vi "Handle Value.vi"(8 "error in (no error)":errorcluster, 10 "Value":string, 11 "Multipart Parser in":refnum<class "Multipart Parser.lvclass">) -> (0 "error out":errorcluster, 3 "Multipart Parser out":refnum<class "Multipart Parser.lvclass">)   [LabVIEW 2020, in "HTTP Utils.lvlib" / "Multipart Parser.lvclass"]
uses:
  Multipart Parser.lvclass
  Multipart Parser.lvclass/Multipart Parser.ctl
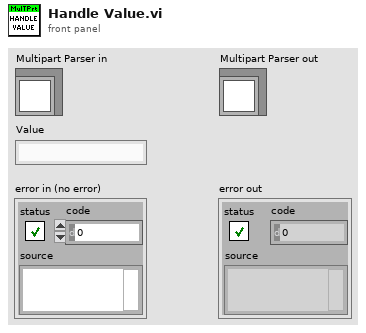
[diagram p1: front panel]
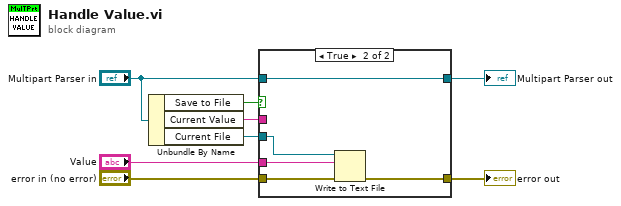
[diagram p0: block diagram]
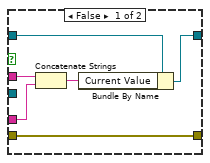
[diagram p2: hidden frame]
diagram:
  n1 = Unbundle By Name("Multipart Parser in") -> ("Save to File"=w7:bool, "Current Value"=w1:string, "Current File"=w5:refnum<file>)
  n2 = case shown="True" w7 {
    tunnel: "error in (no error)" -> [w14 w19]
    tunnel: "Value" -> [w12 w18]
    tunnel: w5 -> [_ w17]
    tunnel: [w14 w16] -> w4
    tunnel: "Multipart Parser in" -> [w11 w15]
    tunnel: [w9 w15] -> w2
    tunnel: w1 -> [w13 _]
    frame False {
      n3 = Concatenate Strings(w13, w12) -> (w10:string)
      n4 = Bundle By Name(cluster=w11, "Current Value"=w10) -> (w9:refnum<class "Multipart Parser.lvclass">)
    }
    frame True {
      n5 = Write to Text File(file (use dialog)=w17, text=w18, error in=w19) -> (error out=w16:errorcluster)  [unwired: 1 in, 2 out]
    }
  }
  "error out" <- w4
  "Multipart Parser out" <- w2
